vi "Query SigGen Frequency Lock.vi"(8 "error in (no error)":errorcluster, 11 "VISA resource":refnum<visa-resource-name>) -> (0 "error out":errorcluster, 2 "Locked":bool, 3 "VISA resource":refnum<visa-resource-name>)   [LabVIEW 2015]
uses:
  <instrlib>/Agilent PSG MXG Series/Agilent PSG MXG Series.lvlib
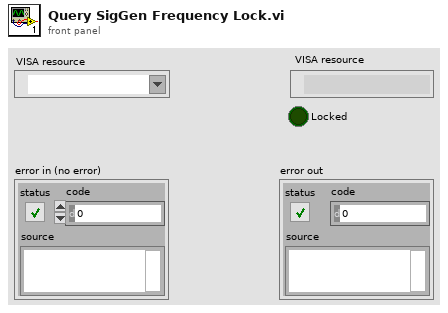
[diagram p1: front panel]
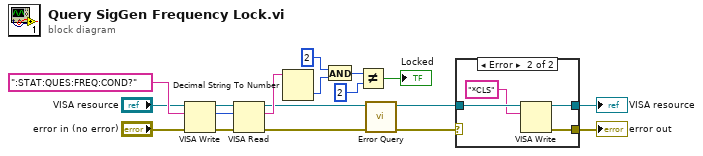
[diagram p0: block diagram]
diagram:
  n1 = VISA Write(VISA resource name="VISA resource", write buffer=":STAT:QUES:FREQ:COND?", error in (no error)="error in (no error)") -> (VISA resource name out=w14:refnum<visa-resource-name>, return count=w18:u32, error out=w13:errorcluster)
  n2 = VISA Read(VISA resource name=w14, byte count=w18, error in (no error)=w13) -> (VISA resource name out=w9:refnum<visa-resource-name>, read buffer=w12:string, error out=w7:errorcluster)  [unwired: 1 out]
  n3 = Decimal String To Number(string=w12) -> (number=w2:i32)  [unwired: 2 in, 1 out]
  n4 = And(x=2, y=w2) -> (x .and. y?=w5:i32)
  n5 = Not Equal?(x=w5, y=2) -> (x != y?=→"Locked":bool)
  n6 = call <instrlib>:"Error Query.vi"("error in (no error)"=w7, "VISA resource name"=w9) -> ("error out"=w1:errorcluster, "VISA resource name out"=w8:refnum<visa-resource-name>)  [unwired: 6 in, 2 out]
  n7 = case shown="Error" w1 {
    selector: w1 -> [w20 _]
    tunnel: [w19 w24] -> w10
    tunnel: w8 -> [w19 w23]
    tunnel: [w20 w22] -> w6
    frame No Error {
    }
    frame Error {
      n8 = VISA Write(VISA resource name=w23, write buffer="*CLS") -> (VISA resource name out=w24:refnum<visa-resource-name>, error out=w22:errorcluster)  [unwired: 1 in, 1 out]
    }
  }
  "VISA resource" <- w10
  "error out" <- w6
